vi "3-lorentzian-heat-response -- analytic derivatives V3.vi"(7 "action":T1, 10 "ω (rad/sec)":dbl=0.1 format="%#_10f", 11 "parameters":dbl[](array[numeric])=[-0.0007412078466363201, -0.0004027798896083045, -0.019859061457473383, -0.00809909374498405, -0.08771864860021968, -0.6888815311338856]) -> (0 "R(ω)":cdb=0.1+0.0i format="%#_10f", 1 "derivatives":cdb[](array[numeric])=[-0.0007412078466363201+0.0i, -0.0004027798896083045+0.0i, -0.019859061457473383+0.0i, -0.00809909374498405+0.0i, -0.08771864860021968+0.0i, -0.6888815311338856+0.0i], 2 "ω out (rad/sec)":dbl=0.1 format="%#_10f", 3 "parameters OUT":dbl[](array[numeric])=[-0.0007412078466363201, -0.0004027798896083045, -0.019859061457473383, -0.00809909374498405, -0.08771864860021968, -0.6888815311338856])   [LabVIEW 2020]
uses:
  3-lorentzian-heat-response action.ctl
panel:
  in  "κ0":dbl(slide)=0.000285 min=0.0 max=0.3 step=1e-06 scale=0.01..10.0 scale format="%#_3p"
  in  "τC":dbl(slide)=0.000285 min=0.0 max=0.3 step=1e-06 scale=0.01..10.0 scale format="%#_3p"
  in  "τN":dbl(slide)=0.000285 min=0.0 max=0.3 step=1e-06 scale=0.01..10.0 scale format="%#_3p"
  in  "τS":dbl(slide)=0.000285 min=0.0 max=0.3 step=1e-06 scale=0.01..10.0 scale format="%#_3p"
  in  "T1":dbl(slide)=0.000285 min=0.0 max=0.3 step=1e-06 scale=0.01..10.0 scale format="%#_3p"
  in  "ζ":dbl(slide)=0.000285 min=0.0 max=0.3 step=1e-06 scale=0.01..10.0 scale format="%#_3p"
  in  "what":cluster{"derivative":T1, "scaling":dbl}[](array[cluster])=[{"derivative"=enum."dζ", "scaling"=1.0}, {"derivative"=enum."dT1", "scaling"=1.0}, {"derivative"=enum."dτS", "scaling"=1.0}, {"derivative"=enum."dτN", "scaling"=1.0}, {"derivative"=enum."dτC", "scaling"=1.0}, {"derivative"=enum."dκ0", "scaling"=0.0}]
  out "d R(ω) / dζ":cdb=-1.0+0.0i
  out "d R(ω) /  dT1":cdb=-1.0+0.0i
  out "d R(ω) /  d τN":cdb=-1.0+0.0i
  out "d R(ω) /  d τS":cdb=-1.0+0.0i
  out "d R(ω) /  d τC":cdb=-1.0+0.0i
  out "d R(ω) /  d κ0":cdb=-1.0+0.0i
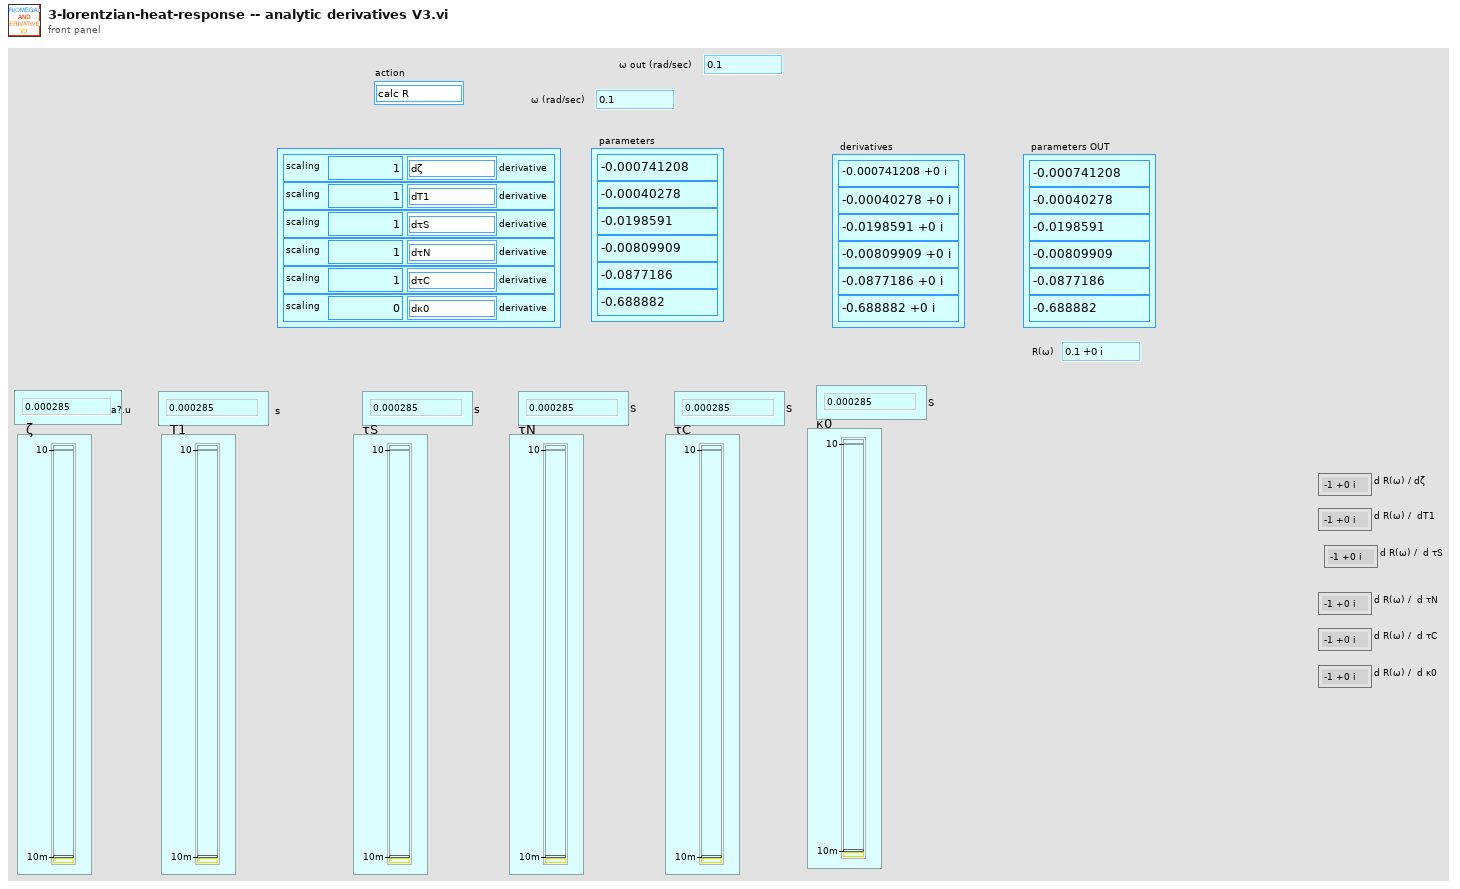
[diagram p1: front panel]
types:
  T1 = typedef "3-lorentzian-heat-response action.ctl" = enum16{"calc R", "create string", "calc m1m2m3", "dζ", "dT1", "dτS", "dτN", "dτC", "d-all", "dκ0", "T(K)", "m1", "m2", "m3", "parse string", "θ (deg)", "B (T)", "onlygrads", "newton", "create emty string"}
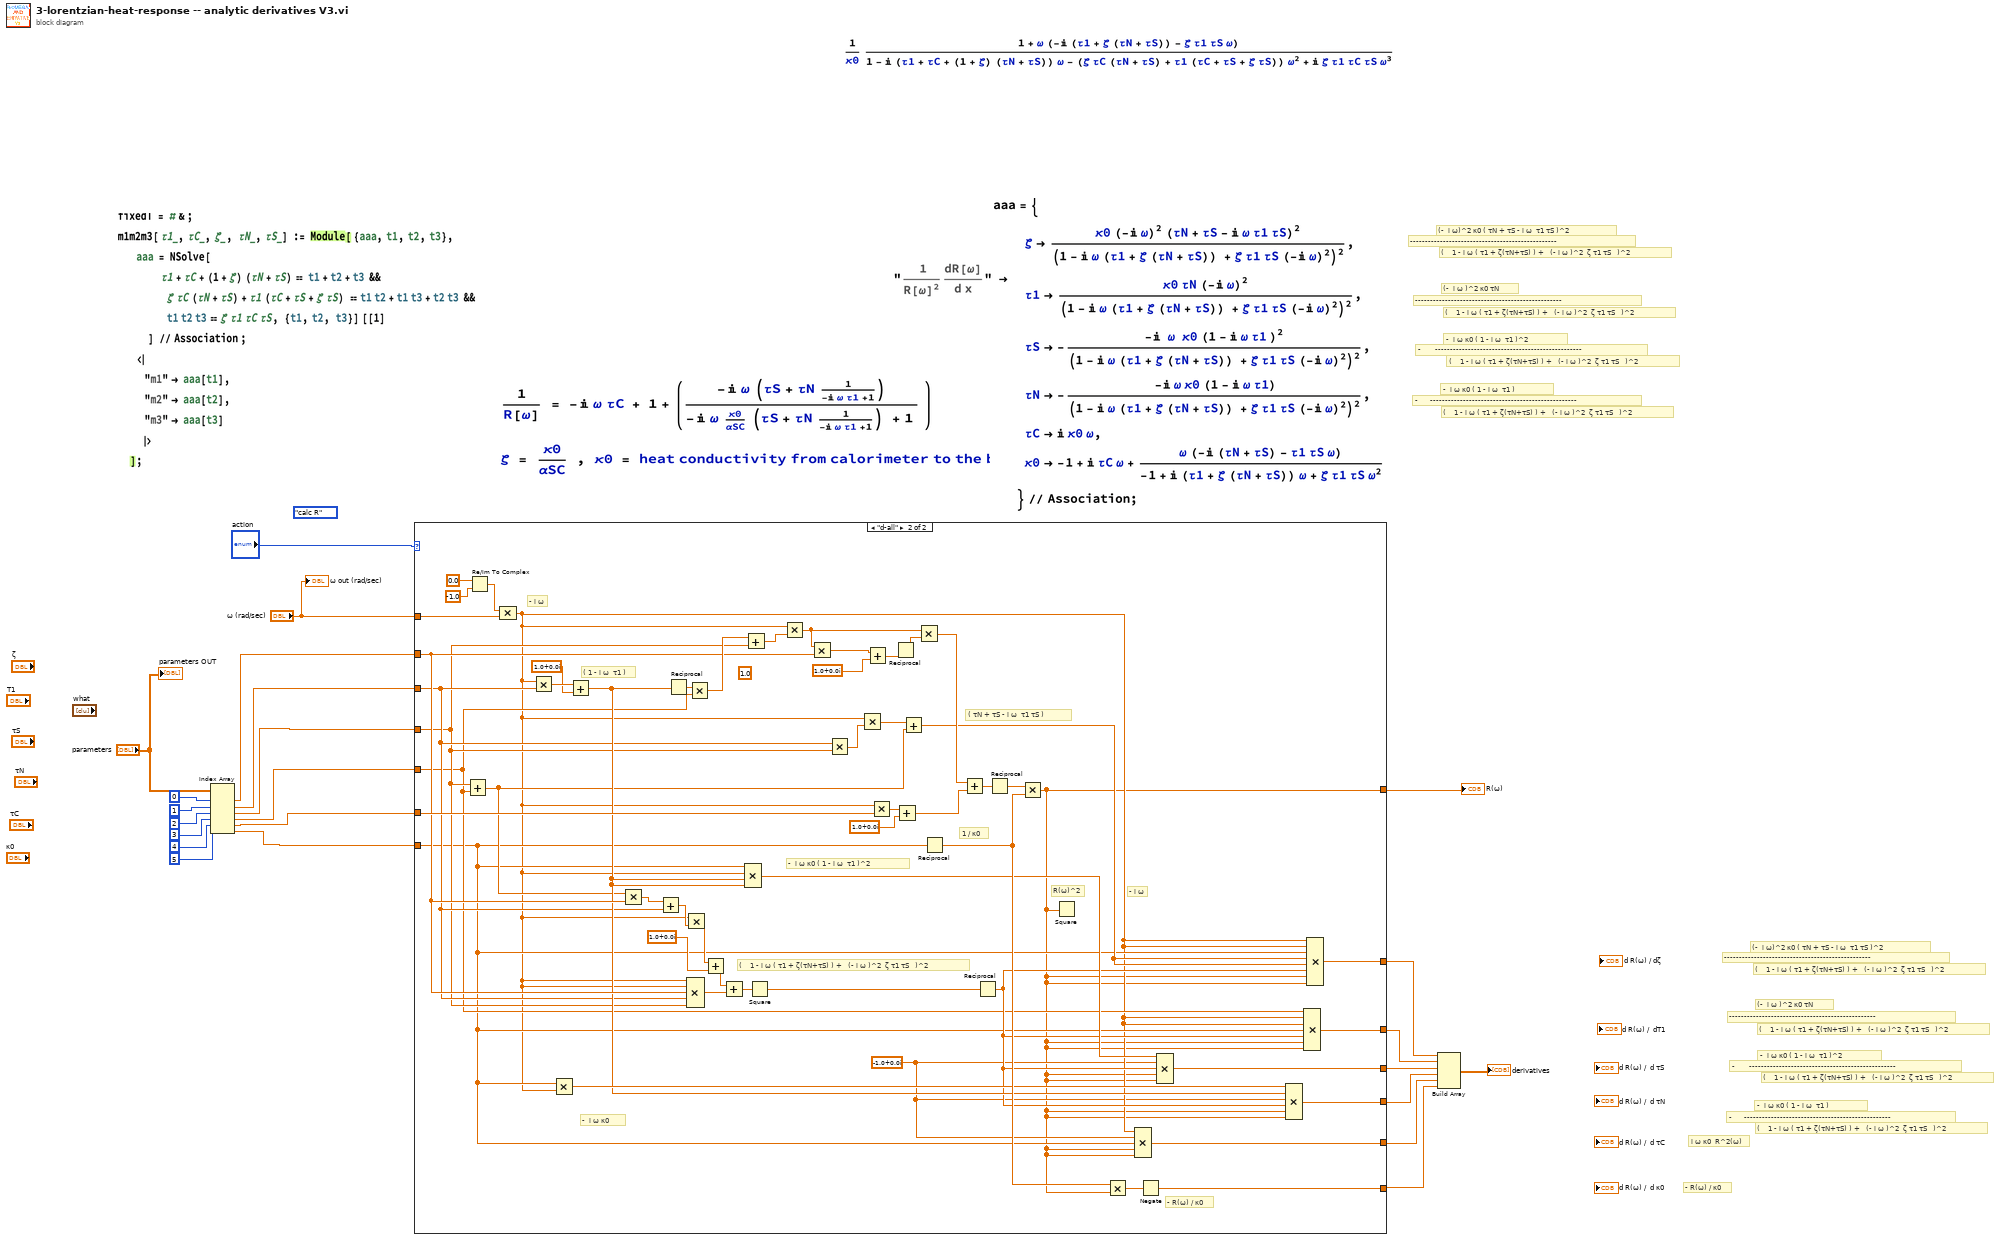
[diagram p0: block diagram]
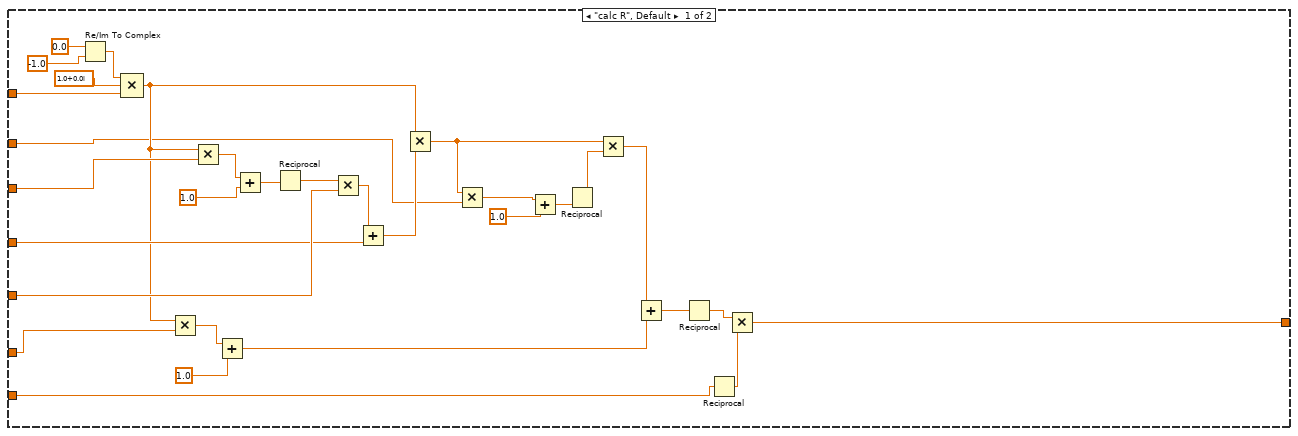
[diagram p2: hidden frame]
diagram:
  (unwired) 3-lorentzian-heat-response_action."calc R" ("action")
  # "-------------------------------------------------"
  # "(-  i ω)^2 κ0 ( τN + τS - i ω  τ1 τS )^2"
  # "(    1 - i ω ( τ1 + ζ(τN+τS) ) +   (- i ω )^2  ζ τ1 τS   )^2"
  # "-------------------------------------------------"
  # "(-  i ω )^2 κ0 τN"
  # "(    1 - i ω ( τ1 + ζ(τN+τS) ) +   (- i ω )^2  ζ τ1 τS   )^2"
  # "-      -------------------------------------------------"
  # "-  i ω κ0 ( 1 - i ω  τ1 )"
  # "(    1 - i ω ( τ1 + ζ(τN+τS) ) +   (- i ω )^2  ζ τ1 τS   )^2"
  # "-       -------------------------------------------------"
  # "-  i ω κ0 ( 1 - i ω  τ1 )^2"
  # "(    1 - i ω ( τ1 + ζ(τN+τS) ) +   (- i ω )^2  ζ τ1 τS   )^2"
  # "-------------------------------------------------"
  # "(-  i ω)^2 κ0 ( τN + τS - i ω  τ1 τS )^2"
  # "(    1 - i ω ( τ1 + ζ(τN+τS) ) +   (- i ω )^2  ζ τ1 τS   )^2"
  # "-------------------------------------------------"
  # "(-  i ω )^2 κ0 τN"
  # "(    1 - i ω ( τ1 + ζ(τN+τS) ) +   (- i ω )^2  ζ τ1 τS   )^2"
  # "-      -------------------------------------------------"
  # "-  i ω κ0 ( 1 - i ω  τ1 )"
  # "(    1 - i ω ( τ1 + ζ(τN+τS) ) +   (- i ω )^2  ζ τ1 τS   )^2"
  # "-       -------------------------------------------------"
  # "-  i ω κ0 ( 1 - i ω  τ1 )^2"
  # "(    1 - i ω ( τ1 + ζ(τN+τS) ) +   (- i ω )^2  ζ τ1 τS   )^2"
  # "i ω κ0  R^2(ω)"
  # "- R(ω) / κ0"
  n1 = Index Array(array="parameters", index #1=0 ("index"), index #2=1 ("index"), index #3=2 ("index"), index #4=3 ("index"), index #5=4 ("index"), index #6=5 ("index")) -> (element #1=w14:dbl, element #2=w13:dbl, element #3=w12:dbl, element #4=w11:dbl, element #5=w10:dbl, element #6=w9:dbl)
  n2 = case shown="\"d-all\"" "action" {
    tunnel: w10 -> [w40 w100]
    tunnel: "ω (rad/sec)" -> [w43 w102]
    tunnel: w13 -> [w42 w67]
    tunnel: w11 -> [w48 w59]
    tunnel: w12 -> [w46 w66]
    tunnel: w14 -> [w36 w78]
    tunnel: [w24 w55] -> w22
    tunnel: w9 -> [w27 w58]
    tunnel: [_ w87] -> w3
    tunnel: [_ w86] -> w4
    tunnel: [_ w72] -> w6
    tunnel: [_ w69] -> w5
    tunnel: [_ w68] -> w7
    tunnel: [_ w60] -> w8
    frame "calc R", Default {
      n3 = Re/Im To Complex(1:-1.0 ("y"), 2:0.0 ("x")) -> (0:w44:cdb)
      n4 = Compound Arithmetic op=MULTIPLY(w44, cdb 1.0+0.0i ("value"), w43) -> (w38:cdb)
      n5 = Multiply(x=w38, y=w40) -> (x*y=w39:cdb)
      n6 = Multiply(x=w38, y=w42) -> (x*y=w41:cdb)
      n7 = Add(x=w39, y=1.0) -> (x+y=w30:cdb)
      n8 = Add(x=w41, y=1.0) -> (x+y=w50:cdb)
      n9 = Reciprocal(x=w50) -> (1/x=w49:cdb)
      n10 = Multiply(x=w49, y=w48) -> (x*y=w47:cdb)
      n11 = Add(x=w47, y=w46) -> (x+y=w37:cdb)
      n12 = Multiply(x=w38, y=w37) -> (x*y=w32:cdb)
      n13 = Multiply(x=w32, y=w36) -> (x*y=w34:cdb)
      n14 = Add(x=w34, y=1.0) -> (x+y=w33:cdb)
      n15 = Reciprocal(x=w33) -> (1/x=w31:cdb)
      n16 = Multiply(x=w32, y=w31) -> (x*y=w29:cdb)
      n17 = Add(x=w29, y=w30) -> (x+y=w28:cdb)
      n18 = Reciprocal(x=w28) -> (1/x=w26:cdb)
      n19 = Reciprocal(x=w27) -> (1/x=w25:dbl)
      n20 = Multiply(x=w26, y=w25) -> (x*y=w24:cdb)
    }
    frame "d-all" {
      w56 = cdb -1.0+0.0i ("value")
      (unwired) 1.0
      # "( τN + τS - i ω  τ1 τS )"
      # "-  i ω κ0"
      # "( 1 - i ω  τ1 )"
      # "(    1 - i ω ( τ1 + ζ(τN+τS) ) +   (- i ω )^2  ζ τ1 τS   )^2"
      # "-  i ω κ0 ( 1 - i ω  τ1 )^2"
      # "- i ω"
      # "1 / κ0"
      # "- R(ω) / κ0"
      # "- i ω"
      # "R(ω)^2"
      n21 = Add(x=w66, y=w59) -> (x+y=w63:dbl)
      n22 = Re/Im To Complex(1:-1.0 ("y"), 2:0.0 ("x")) -> (0:w103:cdb)
      n23 = Compound Arithmetic op=MULTIPLY(w103, w102) -> (w57:cdb)
      n24 = Multiply(x=w57, y=w67) -> (x*y=w101:cdb)
      n25 = Multiply(x=w58, y=w57) -> (x*y=w71:cdb)
      n26 = Add(x=w101, y=cdb 1.0+0.0i ("value")) -> (x+y=w70:cdb)
      n27 = Multiply(x=w63, y=w78) -> (x*y=w82:dbl)
      n28 = Add(x=w82, y=w67) -> (x+y=w81:dbl)
      n29 = Reciprocal(x=w70) -> (1/x=w105:cdb)
      n30 = Multiply(x=w57, y=w81) -> (x*y=w80:cdb)
      n31 = Compound Arithmetic op=MULTIPLY(w57, w57, w78, w67, w66) -> (w76:cdb)
      n32 = Multiply(x=w105, y=w59) -> (x*y=w104:cdb)
      n33 = Add(x=w80, y=cdb 1.0+0.0i ("value")) -> (x+y=w77:cdb)
      n34 = Add(x=w77, y=w76) -> (x+y=w75:cdb)
      n35 = Add(x=w104, y=w66) -> (x+y=w98:cdb)
      n36 = Compound Arithmetic op=MULTIPLY(w58, w57, w70, w70) -> (w74:cdb)
      n37 = Square(x=w75) -> (x^2=w73:cdb)
      n38 = Multiply(x=w57, y=w98) -> (x*y=w95:cdb)
      n39 = Multiply(x=w95, y=w78) -> (x*y=w97:cdb)
      n40 = Multiply(x=w67, y=w66) -> (x*y=w65:dbl)
      n41 = Multiply(x=w57, y=w65) -> (x*y=w64:cdb)
      n42 = Add(x=w97, y=cdb 1.0+0.0i ("value")) -> (x+y=w96:cdb)
      n43 = Multiply(x=w57, y=w100) -> (x*y=w99:cdb)
      n44 = Reciprocal(x=w96) -> (1/x=w94:cdb)
      n45 = Add(x=w99, y=cdb 1.0+0.0i ("value")) -> (x+y=w93:cdb)
      n46 = Add(x=w64, y=w63) -> (x+y=w62:cdb)
      n47 = Multiply(x=w95, y=w94) -> (x*y=w92:cdb)
      n48 = Reciprocal(x=w58) -> (1/x=w89:dbl)
      n49 = Add(x=w92, y=w93) -> (x+y=w91:cdb)
      n50 = Reciprocal(x=w73) -> (1/x=w61:cdb)
      n51 = Reciprocal(x=w91) -> (1/x=w90:cdb)
      n52 = Multiply(x=w90, y=w89) -> (x*y=w55:cdb)
      n53 = Square(x=w55) -> ()  [unwired: 1 out]
      n54 = Multiply(x=w89, y=w55) -> (x*y=w88:cdb)
      n55 = Compound Arithmetic op=MULTIPLY(w57, w56, w58, w55, w55) -> (w86:cdb)
      n56 = Negate(x=w88) -> (-x=w87:cdb)
      n57 = Compound Arithmetic op=MULTIPLY(w74, w56, w61, w55, w55) -> (w72:cdb)
      n58 = Compound Arithmetic op=MULTIPLY(w71, w70, w56, w61, w55, w55) -> (w69:cdb)
      n59 = Compound Arithmetic op=MULTIPLY(w59, w57, w57, w58, w61, w55, w55) -> (w68:cdb)
      n60 = Compound Arithmetic op=MULTIPLY(w57, w57, w58, w62, w62, w61, w55, w55) -> (w60:cdb)
    }
  }
  "R(ω)" <- w22
  n61 = Build Array(w8, w7, w6, w5, w4, w3) -> (→"derivatives":cdb[])
  "parameters OUT" <- "parameters"
  "ω out (rad/sec)" <- "ω (rad/sec)"
